vi "acquire_with_reference_points.vi"() -> ()   [LabVIEW 2013]
uses:
  <vilib>/vision/NI_Vision_Development_Module.lvlib
panel:
  out "Y Co-ordinate (pixels)":dbl[](array[numeric])
  out "X Co ordinate (pixels)":dbl[](array[numeric])
  out "Reference Point in pixels\n (intersection)":cluster{"X":sgl, "Y":sgl} {"Y" format="%.2f"; "X" format="%.2f"}
  out "Circles Data (Circle Detection 1)":T1(array[cluster])
  out "Particle Measurements (Pixels) (Circle Analysis)":dbl[][](array[numeric]) format="%.2f"
  out "Image in":T2(plugin-control)
  in  "Stop":bool
  out "Binary":T2(plugin-control)
  in  "Capture image":bool
  out "Calibrated":T2(plugin-control)
  in  "File Path":path
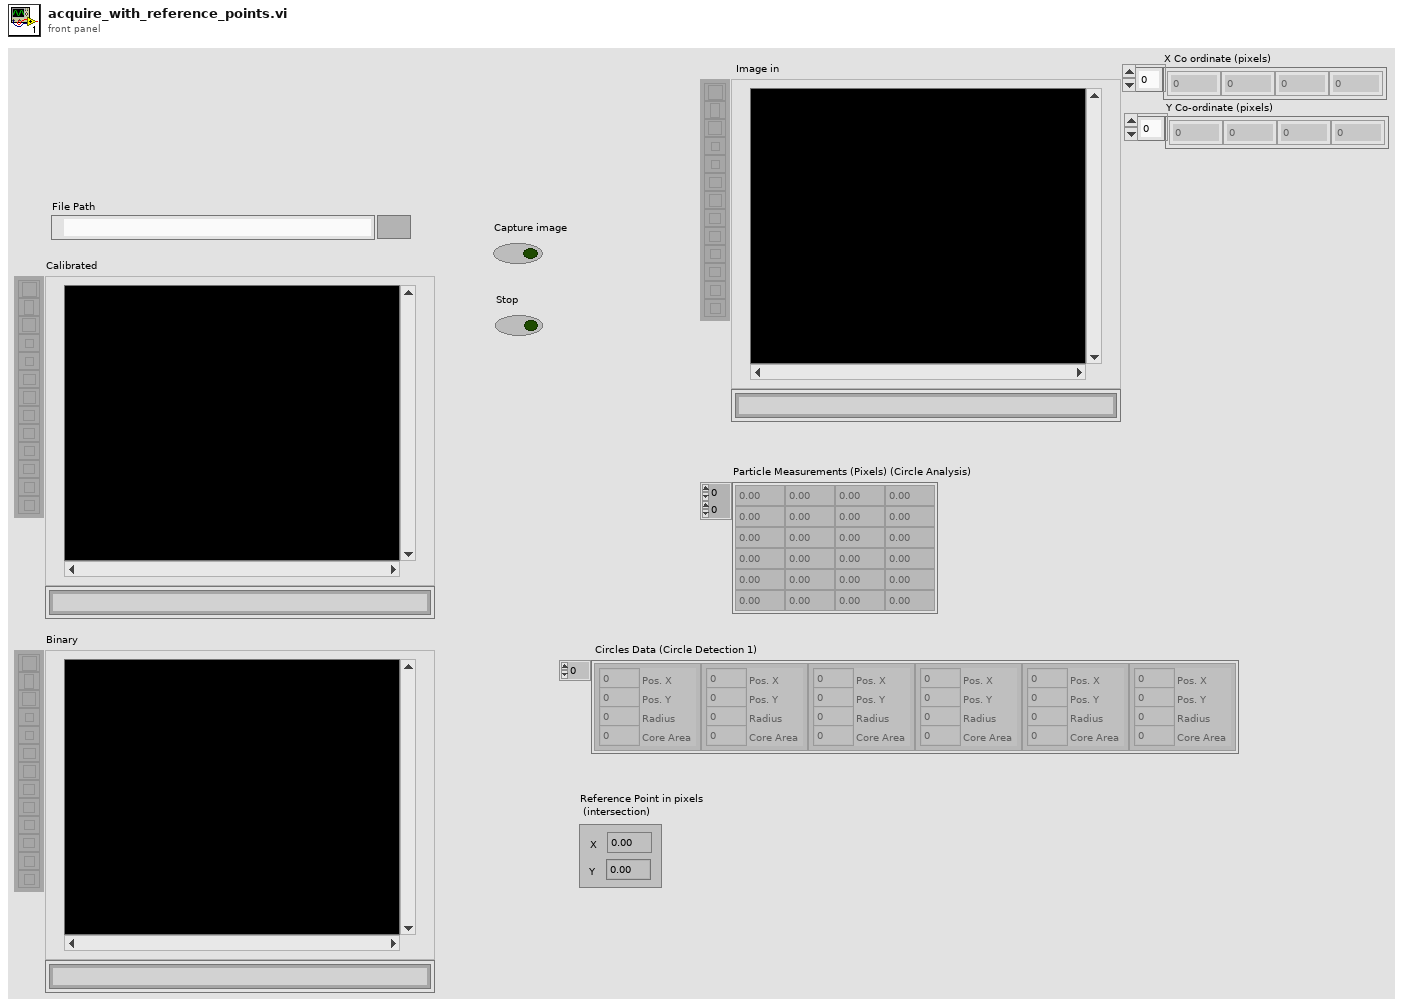
[diagram p1: front panel]
types:
  T1 = cluster{"Pos. X":i32, "Pos. Y":i32, "Radius":i32, "Core Area":i32}[]
  T2 = typedef "IMAQ Image.ctl" = refnum<image>
  T3 = typedef "Image Type" = u32
  T4 = cluster{"Point1 (Pixels)":cluster{"X":sgl, "Y":sgl}, "Point2 (Pixels)":cluster{"X":sgl, "Y":sgl}, "Point1 (Real-World)":cluster{"X":sgl, "Y":sgl}, "Point2 (Real-World)":cluster{"X":sgl, "Y":sgl}, "Angle (Pixel)":dbl, "Angle (Real-World)":dbl, "Score":dbl, "Straightness":dbl, "Average SNR (db)":dbl, "Calibration Valid":bool}
  T5 = cluster{"Point1 (Pixels)":cluster{"X":sgl, "Y":sgl}, "Point2 (Pixels)":cluster{"X":sgl, "Y":sgl}}
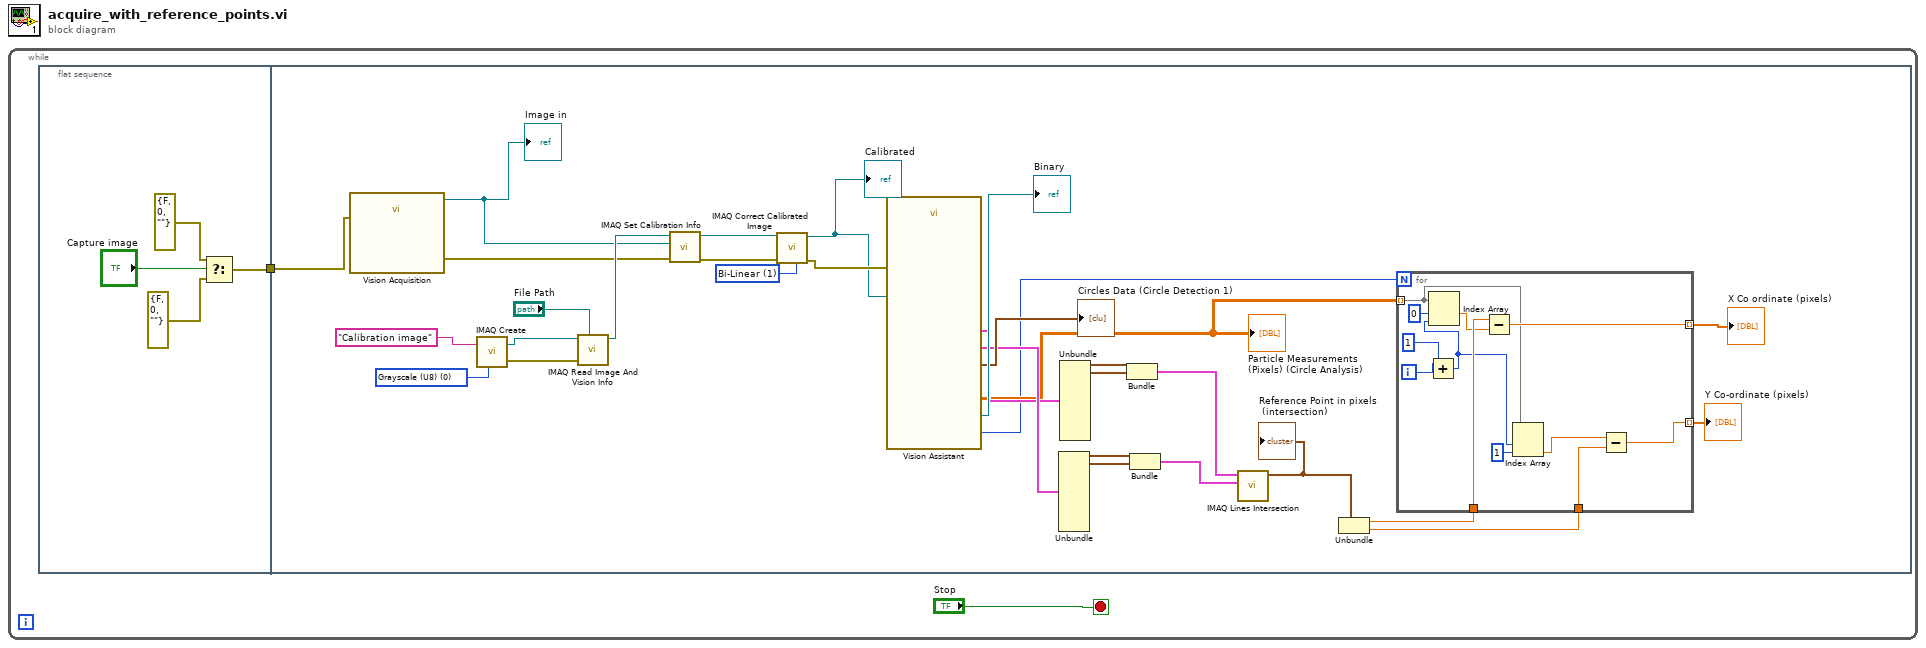
[diagram p0: block diagram]
diagram:
  n1 = while {
    stop <- "Stop" stop-if-true
    n2 = flat-sequence {
      tunnel: [w3] -> w1
      tunnel: w1 -> [w25]
      frame #0 {
        n3 = Select(t=errorcluster {"status"=FALSE, "code"=0, "source"=""} ("error in"), s="Capture image", f=errorcluster {"status"=FALSE, "code"=0, "source"=""} ("error in")) -> (s? t:f=w3:errorcluster)
      }
      frame #1 {
        w32 = T3 0 items=["Grayscale (U8)", "Grayscale (I16)", "Grayscale (SGL)", "Complex (CSG)", "RGB (U32)", "HSL (U32)", "RGB (U64)", "Grayscale (U16)"] ("Image Type")
        w31 = u32 1 items=["Zero Order", "Bi-Linear", "Quadratic", "Cubic Spline"] ("Interpolation Type")
        n4 = call "Vision Acquisition"("error in"=w25) -> ("Image Out"=w27:T2, "error out"=w26:errorcluster)  [unwired: 25 in]
        "Image in" <- w27
        n5 = call "IMAQ Create"("Image Name"="Calibration image", "Image Type"=w32) -> ("New Image"=w37:T2, "error out"=w36:errorcluster)  [unwired: 3 in]
        n6 = call "IMAQ Read Image And Vision Info"("File Path"="File Path", "error in (no error)"=w36, "Image"=w37) -> ("Image Out"=w35:T2)  [unwired: 6 in, 2 out]
        n7 = call "IMAQ Set Calibration Info"("error in (no error)"=w26, "Image Dst"=w27, "Image Src"=w35) -> ("error out"=w30:errorcluster, "Calibrated Image"=w34:T2)  [unwired: 7 in]
        n8 = call "IMAQ Correct Calibrated Image"("Interpolation Type"=w31, "error in (no error)"=w30, "Image Src"=w34) -> ("error out"=w29:errorcluster, "Corrected Image"=w22:T2)  [unwired: 7 in]
        "Calibrated" <- w22
        n9 = call "Vision Assistant"("Image In"=w22, "error in"=w29) -> ("Image Out"=→"Binary":T2, "Particle Measurements (Pixels) (Circle Analysis)"=w12:dbl[][], "Circles Data (Circle Detection 1)"=→"Circles Data (Circle Detection 1)":T1, "Straight Edge (Find Straight Edge 1)"=w17:T4, "Straight Edge (Find Straight Edge 2)"=w21:T4, "Nb Circles (Circle Detection 1)"=w9:i32)  [unwired: 18 in, 2 out]
        "Particle Measurements (Pixels) (Circle Analysis)" <- w12
        n10 = Unbundle(w21) -> ("Point1 (Pixels)"=w20:cluster{"X":sgl, "Y":sgl}, "Point2 (Pixels)"=w19:cluster{"X":sgl, "Y":sgl})  [unwired: 8 out]
        n11 = Unbundle(w17) -> ("Point1 (Pixels)"=w16:cluster{"X":sgl, "Y":sgl}, "Point2 (Pixels)"=w15:cluster{"X":sgl, "Y":sgl})  [unwired: 8 out]
        n12 = Bundle("Point1 (Pixels)"=w16, "Point2 (Pixels)"=w15) -> (w14:T5)  [unwired: 1 in]
        n13 = Bundle("Point1 (Pixels)"=w20, "Point2 (Pixels)"=w19) -> (w18:T5)  [unwired: 1 in]
        n14 = call "IMAQ Lines Intersection"("Line 2"=w18, "Line 1"=w14) -> ("Intersection Point"=w13:cluster{"X":sgl, "Y":sgl})  [unwired: 7 in, 2 out]
        "Reference Point in pixels\n (intersection)" <- w13
        n15 = Unbundle(w13) -> ("X"=w11:sgl, "Y"=w7:sgl)
        n16 = for {
          N: w9 -> [_]
          tunnel: w12 -> [w43] mode=indexing
          tunnel: w11 -> [w49]
          tunnel: [w47] -> w10 mode=indexing
          tunnel: [w38] -> w8 mode=indexing
          tunnel: w7 -> [w40]
          i -> [w45]
          n17 = Add(x=w45, y=1) -> (x+y=w41:i32)
          n18 = Index Array(array=w43, index #1=0 ("index"), index #2=w41) -> (element #1=w48:dbl)  [unwired: 1 out]
          n19 = Subtract(x=w49, y=w48) -> (x-y=w47:dbl)
          n20 = Index Array(array=w43, index #1=w41, index #2=1 ("index")) -> (element #2=w39:dbl)  [unwired: 1 out]
          n21 = Subtract(x=w39, y=w40) -> (x-y=w38:dbl)
        }
        "X Co ordinate (pixels)" <- w10
        "Y Co-ordinate (pixels)" <- w8
      }
    }
  }
